vi "Read Stream.vi"(8 "error in (no error)":errorcluster, 11 "S4 Message Class in":refnum<class "S4 Message Class.lvclass">) -> (0 "error out":errorcluster, 2 "Stream":u8, 3 "S4 Message Class out":refnum<class "S4 Message Class.lvclass">)   [LabVIEW 2020, in "SECS Communication.lvlib" / "S4 Message Class.lvclass"]
uses:
  S4 Message Class.lvclass
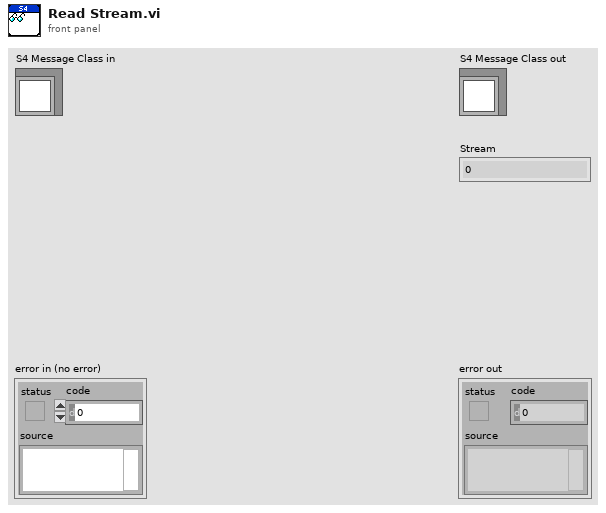
[diagram p1: front panel]
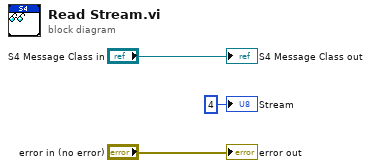
[diagram p0: block diagram]
diagram:
  "error out" <- "error in (no error)"
  "S4 Message Class out" <- "S4 Message Class in"
  "Stream" <- u8 4 ("Stream")
